vi "Main.vi"() -> ()   [LabVIEW 2020, in "Mock Temperature Controller.lvlib"]
uses:
  Mock Temperature Controller.lvlib
  process loops/Instrument Manager/Instrument State.ctl
  process loops/UI Manager/Data Display Loop Data.ctl
  process loops/Logging/Logging Configuration.ctl
  process loops/UI Manager/UI Data.ctl
  process loops/UI Manager/UI Display State.ctl
  Typedefs/System Control Data.ctl
  <vilib>/Utility/error.llb/Error Cluster From Error Code.vi
  <vilib>/ErrorRing/Error Ring.xnode
  support/Message Queue/Message Queue.lvlib
  support/User Event - Stop/User Event - Stop.lvlib
  process loops/Instrument Manager/Instrument Manager.lvlib
  process loops/Acquisition/Acquisition.lvlib
  process loops/Remote Connection Manager/Remote Connection Manager.lvlib
  process loops/Logging/Logging.lvlib
panel:
  in  "Time Interval (sec)":i32=1200
  out "Temperature Graph":cluster{timestamp[], dbl[]}[](graph)
  in  "Config Log Btn":bool
  in  "Sampling rate\n(sec/sample)":dbl=1.0 min=0.1 step=0.1
  in  "Log Data":bool
  in  "Stop Btn":bool=TRUE
  in  "Run Btn":bool
  out "Temperature Ind":dbl format="%.3f °C"
  in  "Setpoint":dbl format="%.3f °C"
  out "VISA resource":refnum<visa-resource-name>
  # "Mock Temperature Controller"
  # "Config"
  # "Instrument Control"
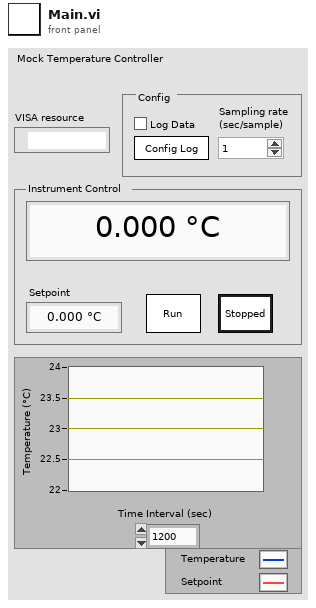
[diagram p1: front panel]
types:
  T1 = typedef "Mock Temperature Controller.lvlib/Data Display Loop Data.ctl" = cluster{"Data Timestamps":timestamp[], "Data Values":dbl[], "Setpoint":dbl[], "Previous Run State":bool}
  T2 = typedef "Mock Temperature Controller.lvlib/Instrument Manager.lvlib/Instrument State.ctl" = cluster{"VISA Resource":refnum<visa-resource-name>, "Setpoint":dbl, "Running":bool, "Running Since":timestamp, "Data Point":cluster{"Time Stamp":timestamp, "Value":dbl}, "Current Temperature":dbl, "Sampling Rate (sec/sample)":dbl}
  T3 = typedef "Mock Temperature Controller.lvlib/Message Queue.lvlib/All Message Queues.ctl" = cluster{"System Control":refnum<queue>, "Instrument":refnum<queue>, "Remote":refnum<queue>, "UI":refnum<queue>, "Acquisition":refnum<queue>, "Logging":refnum<queue>}
  T4 = typedef "Mock Temperature Controller.lvlib/UI Display State.ctl" = enum16{"Shown", "Hidden"}
  T5 = enum8{"Enabled", "Disabled", "Disabled and Grayed Out"}
  T6 = typedef "Mock Temperature Controller.lvlib/UI Data.ctl" = cluster{"VISA Resource Ind":refnum<vi>, "Setpoint Ctl":refnum<vi>, "Run Btn":refnum<vi>, "Stop Btn":refnum<vi>, "Temperature Ind":refnum<vi>, "Log Data":refnum<vi>, "Config Log Btn":refnum<vi>, "Sampling rate\n(sec/sample)":refnum<vi>, "Temperature Graph":refnum<vi>}
  T7 = typedef "Mock Temperature Controller.lvlib/Logging.lvlib/Logging Configuration.ctl" = cluster{"Log Directory Path":path, "Log File Path":path, "Log File Prefix":string, "Log File Extension":string, "File Delimiter":string, "Header Info":string[][], "Channels":string[], "Log Instrument Runs":bool}
  T8 = typedef "Mock Temperature Controller.lvlib/System Control Data.ctl" = cluster{"Example Value <Replace Me>":dbl, "Log Runs":bool, "Clone":bool}
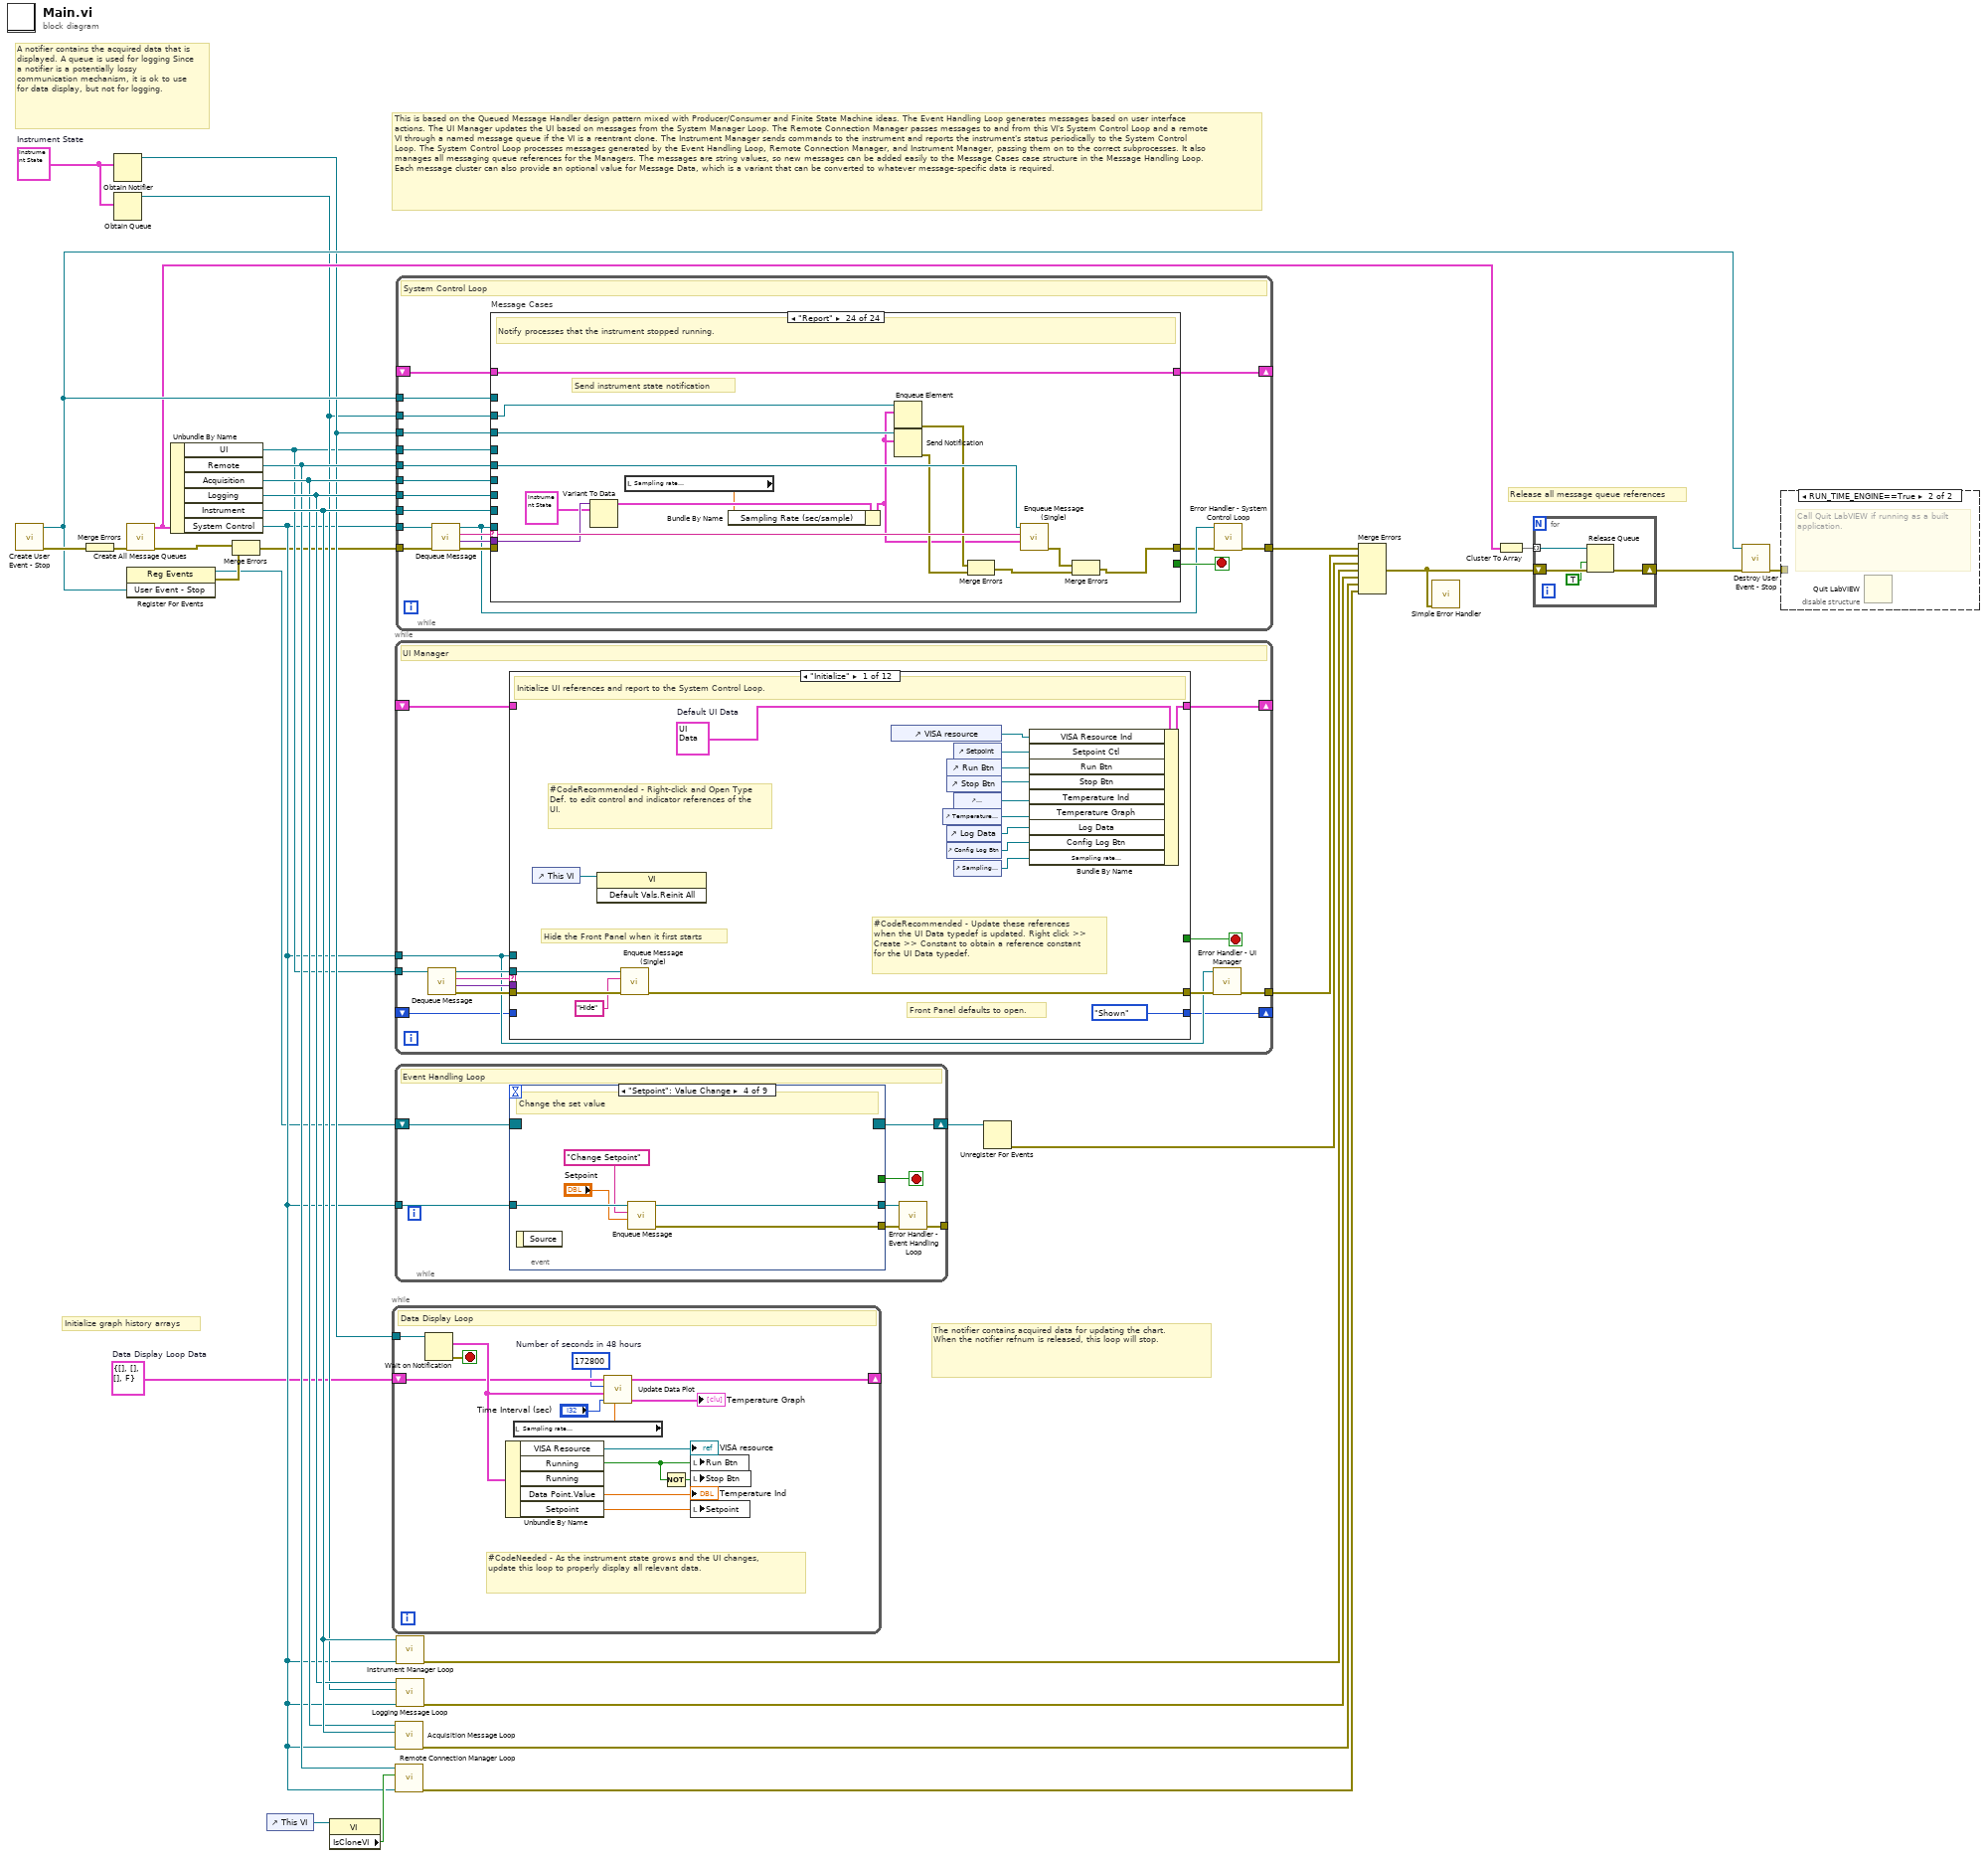
[diagram p0: block diagram]
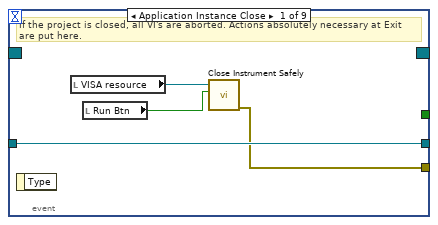
[diagram p2: hidden frame]
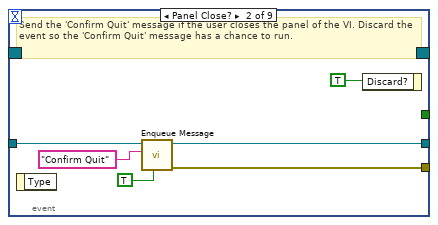
[diagram p3: hidden frame]
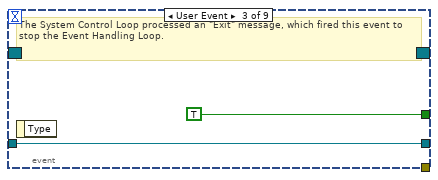
[diagram p4: hidden frame]
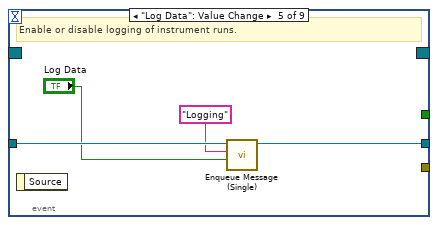
[diagram p5: hidden frame]
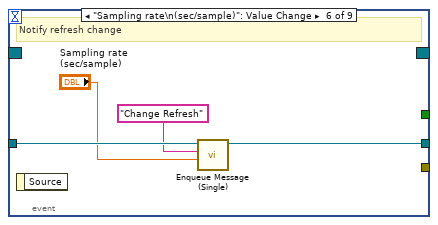
[diagram p6: hidden frame]
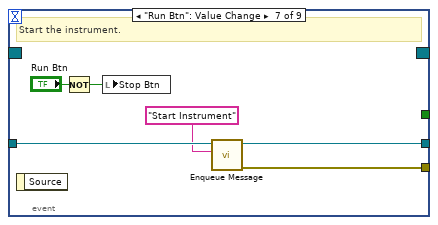
[diagram p7: hidden frame]
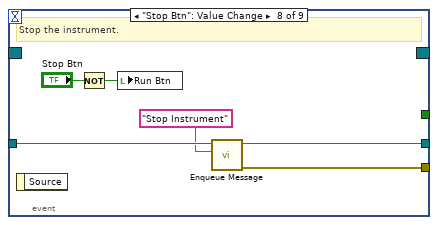
[diagram p8: hidden frame]
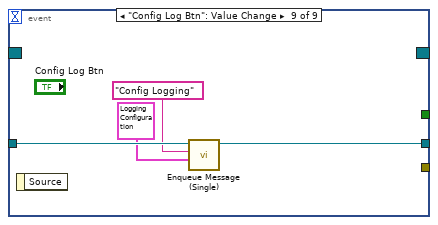
[diagram p9: hidden frame]
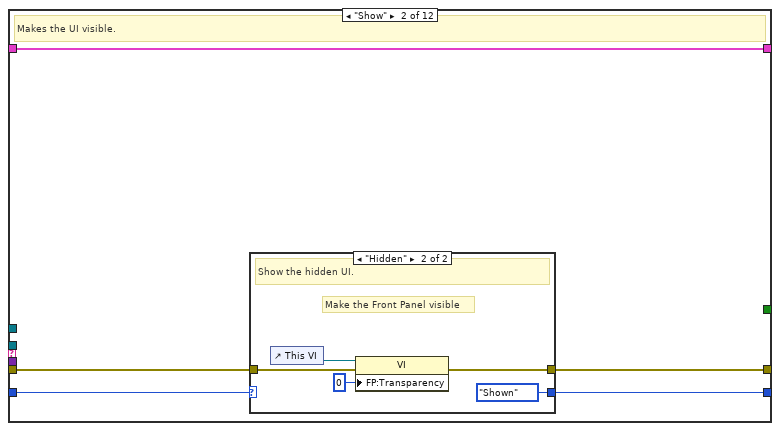
[diagram p10: hidden frame]
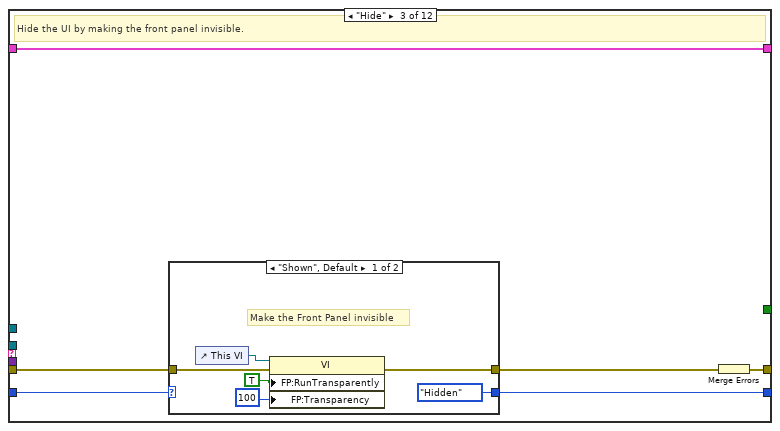
[diagram p12: hidden frame]
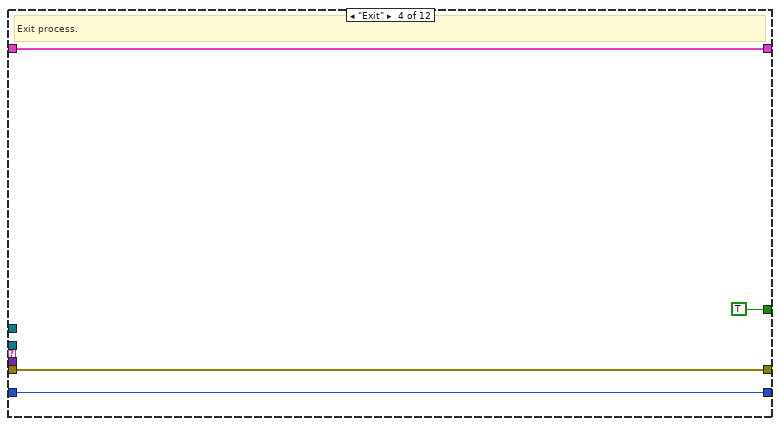
[diagram p14: hidden frame]
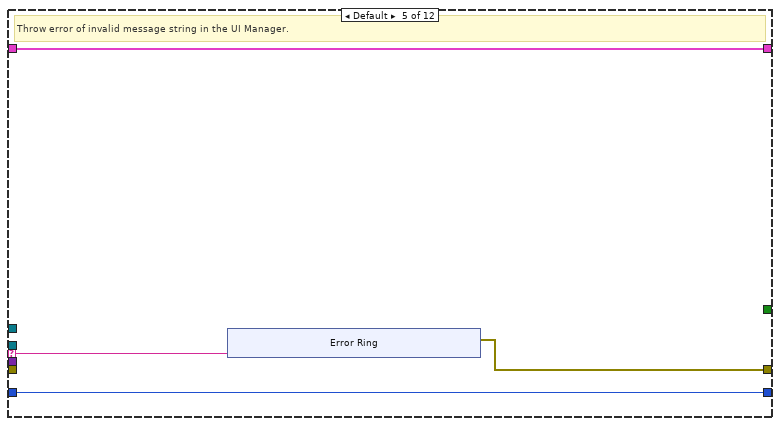
[diagram p15: hidden frame]
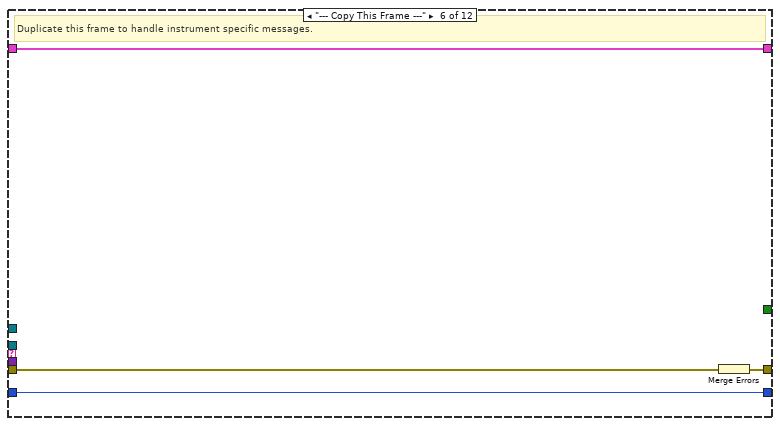
[diagram p16: hidden frame]
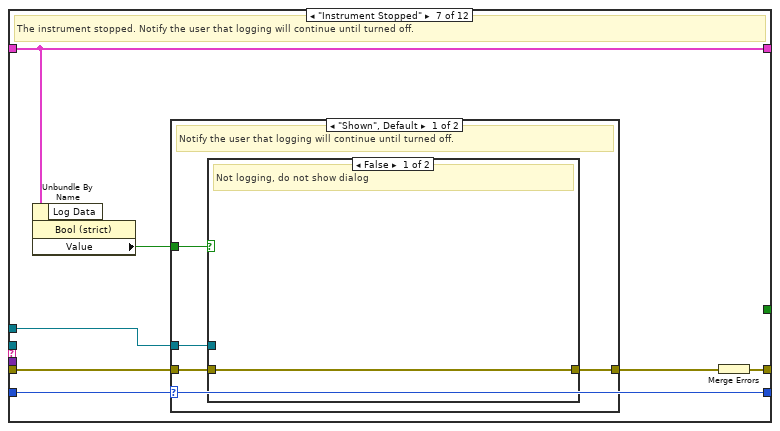
[diagram p17: hidden frame]
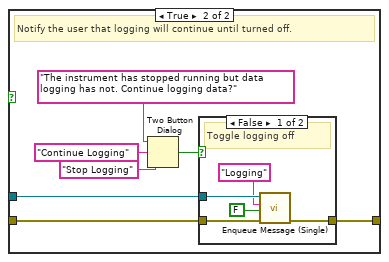
[diagram p18: hidden frame]
diagram:
  w1 = T1 {"Data Timestamps"=[], "Data Values"=[], "Setpoint"=[], "Previous Run State"=FALSE}  # Data Display Loop Data
  w7 = T2 {"VISA Resource"="", "Setpoint"=0.0, "Running"=FALSE, "Running Since"=timestamp(0 s since 1904-01-01), "Data Point"={"Time Stamp"=timestamp(0 s since 1904-01-01), "Value"=0.0}, "Current Temperature"=0.0, "Sampling Rate (sec/sample)"=0.0}  # Instrument State
  # "Initialize graph history arrays"
  # "A notifier contains the acquired data that is displayed. A queue is used for logging Since a notifier is a potentially lossy communication mechanism, it is ok to use for data display, but not for logging."
  # "The notifier contains acquired data for updating the chart. When the notifier refnum is released, this loop will stop."
  # "Release all message queue references"
  # "This is based on the Queued Message Handler design pattern mixed with Producer/Consumer and Finite State Machine ideas. The Event Handling Loop generates messages based on user interface actions. The UI Manager updates the UI based on messages from the System Manager Loop. The Remote Connection Manager passes messages to and from this VI's System Control Loop and a remote VI through a named message queue if the VI is a reentrant clone. The Instrument Manager sends commands to the instrument and reports the instrument's status periodically to the System Control Loop. The System Control Loop processes messages generated by the Event Handling Loop, Remote Connection Manager, and Instrument Manager, passing them on to the correct subprocesses. It also manages all messaging queue references for the Managers. The messages are string values, so new messages can be added easily to the Message Cases case structure in the Message Handling Loop.  Each message cluster can also provide an optional value for Message Data, which is a variant that can be converted to whatever message-specific data is required."
  n1 = call "Create User Event - Stop.vi"() -> ("error out"=w26:errorcluster, "User Event - Stop"=w22:refnum<user-event>)  [unwired: 10 in]
  n2 = Merge Errors(w26) -> (w25:errorcluster)
  n3 = Obtain Notifier(notification data type=w7) -> (notifier out=w8:refnum<notifier>)  [unwired: 3 in, 2 out]
  n4 = Obtain Queue(element data type=w7) -> (queue out=w6:refnum<queue>)  [unwired: 4 in, 2 out]
  n5 = call "Create All Message Queues.vi"("error in (no error)"=w25) -> ("error out"=w28:errorcluster, "Message Queues out"=w11:T3)  [unwired: 9 in]
  n6 = register-events(w22) -> (reference out=w2:refnum<event-registration>, error out=w13:errorcluster)  [unwired: 2 in]
  n7 = Unbundle By Name(w11) -> ("UI"=w5:refnum<queue>, "Remote"=w29:refnum<queue>, "Acquisition"=w30:refnum<queue>, "Logging"=w31:refnum<queue>, "Instrument"=w32:refnum<queue>, "System Control"=w4:refnum<queue>)
  n8 = Merge Errors(w28, w13) -> (w3:errorcluster)
  n9 = control-ref of="This VI"() -> (w21:refnum<vi>)
  n10 = property class="VI"(reference=w21) -> ("IsCloneVI"=w20:bool)  [unwired: 1 in, 2 out]
  n11 = while "Data Display Loop" {
    tunnel: w8 -> [w46]
    shift-right: [w36] -> _
    shift-left: w1 -> [w37]
    stop <- w45 stop-if-true
    w33 = 172800  # Number of seconds in 48 hours
    # "#CodeNeeded - As the instrument state grows and the UI changes, update this loop to properly display all relevant data."
    # "Data Display Loop"
    n12 = Wait on Notification(notifier=w46) -> (notification=w38:T2, error out=w45:errorcluster)  [unwired: 3 in, 2 out]
    n13 = Unbundle By Name(w38) -> ("VISA Resource"=→"VISA resource":refnum<visa-resource-name>, "Running"=w43:bool, "Data Point.Value"=→"Temperature Ind":dbl, "Setpoint"=w40:dbl)  [unwired: 1 out]
    n14 = local read "Sampling rate\n(sec/sample)"() -> (w34:dbl)
    n15 = call "Update Data Plot.vi"("Sample Rate (sec/sample)"=w34, "Time interval (s)"="Time Interval (sec)", "Instrument State"=w38, "History length"=w33, "Graph History Arrays in"=w37) -> ("Updated Plot History"=→"Temperature Graph":cluster{timestamp[], dbl[]}[], "Graph History Arrays out"=w36:T1)  [unwired: 5 in]
    n16 = Not(x=w43) -> (.not. x?=w42:bool)
    n17 = local write "Run Btn"(w43) -> ()
    n18 = local write "Stop Btn"(w42) -> ()
    n19 = local write "Setpoint"(w40) -> ()
  }
  n20 = while {
    tunnel: w5 -> [w59]
    tunnel: w4 -> [w50]
    tunnel: [w51] -> w19
    shift-right: [w54] -> _
    shift-left: _ -> [w53]
    shift-right: [w48] -> _
    shift-left: _ -> [w47]
    stop <- w49 stop-if-true
    # "UI Manager"
    n21 = call "Dequeue Message.vi"("Message Queue"=w59) -> ("error out"=w57:errorcluster, "Message Data"=w55:variant, "Message"=w56:string, "dup Message Queue"=w58:refnum<queue>)  [unwired: 7 in]
    n22 = case shown="\"Initialize\"" w56 {
      selector: w56 -> [_ _ _ _ w110 _ _ _ _ _ _ _]
      tunnel: w58 -> [w67 _ _ _ _ _ _ _ _ _ _ _]
      tunnel: w57 -> [w73 w80 w92 w106 _ w119 w127 w155 w163 w171 w182 w193]
      tunnel: w55 -> [_ _ _ _ _ _ _ _ _ w170 w180 w191]
      tunnel: w50 -> [_ _ _ _ _ _ w125 _ _ _ _ _]
      tunnel: [w68 w79 w93 w106 w109 w120 w129 w156 w164 w172 w183 w194] -> w52
      tunnel: [w75 w81 w94 w105 w108 w121 w124 w151 w157 w166 w174 w185] -> w54
      tunnel: w53 -> [_ w81 w94 w105 w108 w121 w124 w151 w157 w166 w174 w185]
      tunnel: [_ _ _ TRUE _ _ _ _ _ _ _ _] -> w49
      tunnel: w47 -> [_ w78 w90 w103 w107 w118 w128 w154 w162 w168 w175 w186]
      tunnel: [UI_Display_State."Shown" ("UI Display State") w77 w89 w103 w107 w118 w128 w154 w162 w168 w175 w186] -> w48
      frame "Initialize" {
        w76 = T6 {"VISA Resource Ind"=refnum, "Setpoint Ctl"=refnum, "Run Btn"=refnum, "Stop Btn"=refnum, "Temperature Ind"=refnum, "Log Data"=refnum, "Config Log Btn"=refnum, "Sampling rate\n(sec/sample)"=refnum, "Temperature Graph"=refnum}  # Default UI Data
        # "Front Panel defaults to open."
        # "Hide the Front Panel when it first starts"
        # "#CodeRecommended - Update these references when the UI Data typedef is updated. Right click >> Create >> Constant to obtain a reference constant for the UI Data typedef."
        # "#CodeRecommended - Right-click and Open Type Def. to edit control and indicator references of the UI."
        # "Initialize UI references and report to the System Control Loop."
        n23 = control-ref of="This VI"() -> (w60:refnum<vi>)
        n24 = invoke class="VI" method="Default Vals.Reinit All"(reference=w60) -> ()  [unwired: 2 in, 3 out]
        n25 = call "Enqueue Message (Single).vi"("error in (no error)"=w73, "Message"="Hide", "Message Queue"=w67) -> ("error out"=w68:errorcluster)  [unwired: 7 in, 1 out]
        n26 = control-ref of="VISA resource"() -> (w72:refnum<vi>)
        n27 = control-ref of="Temperature Graph"() -> (w64:refnum<vi>)
        n28 = control-ref of="Run Btn"() -> (w70:refnum<vi>)
        n29 = control-ref of="Stop Btn"() -> (w71:refnum<vi>)
        n30 = control-ref of="Log Data"() -> (w63:refnum<vi>)
        n31 = control-ref of="Config Log Btn"() -> (w62:refnum<vi>)
        n32 = control-ref of="Setpoint"() -> (w74:refnum<vi>)
        n33 = control-ref of="Temperature Ind"() -> (w69:refnum<vi>)
        n34 = control-ref of="Sampling rate (sec/sample)"() -> (w61:refnum<vi>)
        n35 = Bundle By Name(cluster=w76, "VISA Resource Ind"=w72, "Setpoint Ctl"=w74, "Run Btn"=w70, "Stop Btn"=w71, "Temperature Ind"=w69, "Temperature Graph"=w64, "Log Data"=w63, "Config Log Btn"=w62, "Sampling rate\n(sec/sample)"=w61) -> (w75:T6)
      }
      frame "Show" {
        # "Makes the UI visible."
        n36 = case shown="\"Hidden\"" w78 {
          selector: w78 -> [w83 _]
          tunnel: w80 -> [w82 w88]
          tunnel: [w82 w86] -> w79
          tunnel: [w83 UI_Display_State."Shown" ("UI Display State")] -> w77
          frame "Shown", Default {
            # "Do nothing if UI is already shown."
          }
          frame "Hidden" {
            # "Make the Front Panel visible"
            # "Show the hidden UI."
            n37 = control-ref of="This VI"() -> (w87:refnum<vi>)
            n38 = property class="VI"(reference=w87, error in=w88, "FP:Transparency"=u8 0 ("Front Panel Window:Transparency")) -> (error out=w86:errorcluster)  [unwired: 1 out]
          }
        }
      }
      frame "Hide" {
        # "Hide the UI by making the front panel invisible."
        n39 = case shown="\"Shown\", Default" w90 {
          selector: w90 -> [_ w102]
          tunnel: w92 -> [w97 w101]
          tunnel: [w96 w101] -> w91
          tunnel: [UI_Display_State."Hidden" ("UI Display State") w102] -> w89
          frame "Shown", Default {
            # "Make the Front Panel invisible"
            n40 = control-ref of="This VI"() -> (w100:refnum<vi>)
            n41 = property class="VI"(reference=w100, error in=w97, "FP:RunTransparently"=TRUE ("Front Panel Window:Run VI Transparently"), "FP:Transparency"=u8 100 ("Front Panel Window:Transparency")) -> (error out=w96:errorcluster)  [unwired: 1 out]
          }
          frame "Hidden" {
          }
        }
        n42 = Merge Errors(w91) -> (w93:errorcluster)
      }
      frame "Exit" {
        # "Exit process."
      }
      frame Default {
        # "Throw error of invalid message string in the UI Manager."
        n43 = xnode "Error Ring"("parameter 0"=w110) -> ("error out"=w109:errorcluster)
      }
      frame "--- Copy This Frame ---" {
        # "Duplicate this frame to handle instrument specific messages."
        n44 = Merge Errors(w119) -> (w120:errorcluster)
      }
      frame "Instrument Stopped" {
        # "The instrument stopped. Notify the user that logging will continue until turned off."
        n45 = Unbundle By Name(w124) -> ("Log Data"=w123:refnum<vi>)
        n46 = property class="Bool (strict)"(reference=w123) -> ("Value"=w122:bool)  [unwired: 1 in, 2 out]
        n47 = case shown="\"Shown\", Default" w128 {
          tunnel: w127 -> [w133 w148]
          tunnel: [w132 w148] -> w126
          tunnel: w125 -> [w131 _]
          tunnel: w122 -> [w130 _]
          frame "Shown", Default {
            # "Notify the user that logging will continue until turned off."
            n48 = case shown="False" w130 {
              tunnel: w133 -> [w134 w137]
              tunnel: [w134 w136] -> w132
              tunnel: w131 -> [_ w135]
              frame False {
                # "Not logging, do not show dialog"
              }
              frame True {
                # "Notify the user that logging will continue until turned off."
                n49 = Two Button Dialog(message="The instrument has stopped running but data logging has not. Continue logging data?", 1:"Stop Logging" ("F button name (\"Cancel\")"), 2:"Continue Logging" ("T button name (\"OK\")")) -> (T button?=w138:bool)
                n50 = case shown="False" w138 {
                  tunnel: w137 -> [w146 w147]
                  tunnel: [w145 w147] -> w136
                  tunnel: w135 -> [w144 _]
                  frame False {
                    # "Toggle logging off"
                    n51 = call "Enqueue Message (Single).vi"("error in (no error)"=w146, "Message Data"=FALSE, "Message"="Logging", "Message Queue"=w144) -> ("error out"=w145:errorcluster)  [unwired: 6 in, 1 out]
                  }
                  frame True {
                    # "Continues logging. Do nothing more"
                  }
                }
              }
            }
          }
          frame "Hidden" {
            # "Hidden, do not show dialog"
          }
        }
        n52 = Merge Errors(w126) -> (w129:errorcluster)
      }
      frame "Logging Started" {
        # "Indicate that logging started."
        n53 = Unbundle By Name(w151) -> ("Log Data"=w153:refnum<vi>)
        n54 = property class="Bool (strict)"(reference=w153, "Value"=TRUE ("Log Data")) -> ()  [unwired: 1 in, 2 out]
        n55 = Unbundle By Name(w151) -> ("Config Log Btn"=w150:refnum<vi>)
        n56 = property class="Bool"(reference=w150, "DisabledEnum"=T5."Disabled and Grayed Out" ("Disabled")) -> ()  [unwired: 1 in, 2 out]
        n57 = Merge Errors(w155) -> (w156:errorcluster)
      }
      frame "Logging Stopped" {
        # "Indicate that logging stopped."
        n58 = Unbundle By Name(w157) -> ("Log Data"=w161:refnum<vi>)
        n59 = property class="Bool (strict)"(reference=w161, "Value"=FALSE ("Log Data")) -> ()  [unwired: 1 in, 2 out]
        n60 = Unbundle By Name(w157) -> ("Config Log Btn"=w159:refnum<vi>)
        n61 = property class="Bool"(reference=w159, "DisabledEnum"=T5."Enabled" ("Disabled")) -> ()  [unwired: 1 in, 2 out]
        n62 = Merge Errors(w163) -> (w164:errorcluster)
      }
      frame "Change Refresh" {
        # "Update sample rate multiplier in the UI data chart and config indicator."
        n63 = Unbundle By Name(w166) -> ("Sampling rate\n(sec/sample)"=w167:refnum<vi>)
        n64 = Variant To Data(type=0.0, Variant=w170) -> (data=w165:dbl)  [unwired: 1 in, 1 out]
        n65 = property class="DigNum (strict)"(reference=w167, "Value"=w165) -> ()  [unwired: 1 in, 2 out]
        n66 = Merge Errors(w171) -> (w172:errorcluster)
      }
      frame "Display Units - Temperature Ind" {
        # "#CodeRecommended - If this format string is changed, update it on the front panel indicator as well."
        # "Change the units of the display."
        n67 = Variant To Data(type="", Variant=w180) -> (data=w178:string)  [unwired: 1 in, 1 out]
        n68 = call <vilib>:"Space Constant.vi"() -> ("String"=w179:string)
        n69 = Concatenate Strings("%.3f" ("string"), w179, w178) -> (w176:string)
        n70 = Unbundle By Name(w174) -> ("Temperature Ind"=w173:refnum<vi>)
        n71 = property on="Property Node" class="DigNum (strict)"(reference=w173, "FormatString"=w176) -> ()  [unwired: 1 in, 2 out]
        n72 = Merge Errors(w182) -> (w183:errorcluster)
      }
      frame "Display Units - Setpoint" {
        # "#CodeRecommended - If this format string is changed, update it on the front panel indicator as well."
        # "Change the units of the setpoint display."
        n73 = Variant To Data(type="", Variant=w191) -> (data=w189:string)  [unwired: 1 in, 1 out]
        n74 = call <vilib>:"Space Constant.vi"() -> ("String"=w190:string)
        n75 = Concatenate Strings("%.3f" ("string"), w190, w189) -> (w187:string)
        n76 = Unbundle By Name(w185) -> ("Setpoint Ctl"=w184:refnum<vi>)
        n77 = property on="Property Node" class="DigNum (strict)"(reference=w184, "FormatString"=w187) -> ()  [unwired: 1 in, 2 out]
        n78 = Merge Errors(w193) -> (w194:errorcluster)
      }
    }
    n79 = call "Error Handler - UI Manager.vi"("error in (no error)"=w52, "Message Queue"=w50) -> ("dup error in"=w51:errorcluster)  [unwired: 8 in, 1 out]
  }
  n80 = while {
    tunnel: w4 -> [w201]
    shift-right: [w199] -> w23
    shift-left: w2 -> [w200]
    tunnel: [w195] -> _
    stop <- w197 stop-if-true
    # "Event Handling Loop"
    n81 = event shown="[3] \"Setpoint\": Value Change" {
      selector: w200 -> [_ _ _ _ _ _ _ _ _]
      dyn-events: [_ _ _ _ _ _ _ _ _] -> w199
      timeout: _ -> [_ _ _ _ _ _ _ _ _]
      tunnel: [_ _ TRUE ("Discard?") _ _ _ _ _ _] -> w197
      tunnel: w201 -> [w205 w210 w213 w218 w222 w226 w232 w238 w242]
      tunnel: [w204 w209 _ w215 _ _ w230 w236 _] -> w198
      tunnel: [w205 w208 w213 w217 w221 w225 w231 w237 w241] -> w196
      event Application Instance Close {
        # "If the project is closed, all VI's are aborted. Actions absolutely necessary at Exit are put here."
        n82 = event-data() -> ()  [unwired: 1 in, 1 out]
        n83 = local read "VISA resource"() -> (w203:refnum<visa-resource-name>)
        n84 = local read "Run Btn"() -> (w202:bool)
        n85 = call "Close Instrument Safely.vi"("Running (F)"=w202, "VISA Refnum in"=w203) -> ("error out"=w204:errorcluster)  [unwired: 9 in]
      }
      event Panel Close? {
        # "Send the 'Confirm Quit' message if the user closes the panel of the VI. Discard the event so the 'Confirm Quit' message has a chance to run."
        n86 = event-data() -> ()  [unwired: 1 in, 1 out]
        n87 = call-poly "Enqueue Message.vi"("Priority Message? (F)"=TRUE, "Message"="Confirm Quit", "Message Queue"=w210) -> ("error out"=w209:errorcluster, "dup Message Queue"=w208:refnum<queue>)  [unwired: 7 in]
        n88 = event-data("Discard?"=TRUE) -> ()  [unwired: 1 in, 1 out]
      }
      event User Event {
        # "The System Control Loop processed an \"Exit\" message, which fired this event to stop the Event Handling Loop."
        n89 = event-data() -> ()  [unwired: 1 in, 1 out]
      }
      event "Setpoint": Value Change {
        # "Change the set value"
        n90 = event-data() -> ()  [unwired: 1 in, 1 out]
        n91 = call-poly "Enqueue Message.vi"("Message Data"="Setpoint", "Message"="Change Setpoint", "Message Queue"=w218) -> ("error out"=w215:errorcluster, "dup Message Queue"=w217:refnum<queue>)  [unwired: 7 in]
      }
      event "Log Data": Value Change {
        # "Enable or disable logging of instrument runs."
        n92 = event-data() -> ()  [unwired: 1 in, 1 out]
        n93 = call "Enqueue Message (Single).vi"("Message Data"="Log Data", "Message"="Logging", "Message Queue"=w222) -> ("dup Message Queue"=w221:refnum<queue>)  [unwired: 7 in, 1 out]
      }
      event "Sampling rate\n(sec/sample)": Value Change {
        # "Notify refresh change"
        n94 = event-data() -> ()  [unwired: 1 in, 1 out]
        n95 = call "Enqueue Message (Single).vi"("Message Data"="Sampling rate\n(sec/sample)", "Message"="Change Refresh", "Message Queue"=w226) -> ("dup Message Queue"=w225:refnum<queue>)  [unwired: 7 in, 1 out]
      }
      event "Run Btn": Value Change {
        # "Start the instrument."
        n96 = event-data() -> ()  [unwired: 1 in, 1 out]
        n97 = Not(x="Run Btn") -> (.not. x?=w227:bool)
        n98 = local write "Stop Btn"(w227) -> ()
        n99 = call-poly "Enqueue Message.vi"("Message"="Start Instrument", "Message Queue"=w232) -> ("error out"=w230:errorcluster, "dup Message Queue"=w231:refnum<queue>)  [unwired: 8 in]
      }
      event "Stop Btn": Value Change {
        # "Stop the instrument."
        n100 = event-data() -> ()  [unwired: 1 in, 1 out]
        n101 = Not(x="Stop Btn") -> (.not. x?=w233:bool)
        n102 = local write "Run Btn"(w233) -> ()
        n103 = call-poly "Enqueue Message.vi"("Message"="Stop Instrument", "Message Queue"=w238) -> ("error out"=w236:errorcluster, "dup Message Queue"=w237:refnum<queue>)  [unwired: 8 in]
      }
      event "Config Log Btn": Value Change {
        n104 = event-data() -> ()  [unwired: 1 in, 1 out]
        n105 = call "Enqueue Message (Single).vi"("Message Data"=T7 {"Log Directory Path"=path "", "Log File Path"=path "", "Log File Prefix"="Experiment", "Log File Extension"="csv", "File Delimiter"=",", "Header Info"=[], "Channels"=[], "Log Instrument Runs"=FALSE} ("Logging Configuration"), "Message"="Config Logging", "Message Queue"=w242) -> ("dup Message Queue"=w241:refnum<queue>)  [unwired: 7 in, 1 out]
      }
    }
    n106 = call "Error Handler - Event Handling Loop.vi"("error in (no error)"=w198, "Message Queue"=w196) -> ("dup error in"=w195:errorcluster)  [unwired: 8 in, 1 out]
  }
  n107 = call "Acquisition Message Loop.vi"("System Control"=w4, "Instrument Manager"=w32, "Acquisition"=w30) -> ("error out"=w15:errorcluster)  [unwired: 8 in]
  n108 = call "Remote Connection Manager Loop.vi"("System Control"=w4, "IsCloneVI (false)"=w20, "RCM Queue"=w29) -> ("error out"=w14:errorcluster)  [unwired: 8 in]
  n109 = while {
    tunnel: w4 -> [w253]
    shift-right: [w260] -> _
    shift-left: _ -> [w261]
    tunnel: w22 -> [w258]
    tunnel: w3 -> [w257]
    tunnel: [w251] -> w27
    tunnel: w32 -> [w249]
    tunnel: w29 -> [w248]
    tunnel: w5 -> [w247]
    tunnel: w30 -> [w246]
    tunnel: w31 -> [w245]
    tunnel: w8 -> [w244]
    tunnel: w6 -> [w243]
    stop <- w259 stop-if-true
    # "System Control Loop"
    n110 = call "Dequeue Message.vi"("error in (no error)"=w257, "Message Queue"=w253) -> ("error out"=w256:errorcluster, "Message Data"=w254:variant, "Message"=w255:string, "dup Message Queue"=w252:refnum<queue>)  [unwired: 6 in]
    n111 = case "Message Cases" shown="\"Report\"" w255 {
      selector: w255 -> [_ _ _ w303 w316 w327 w345 w359 w365 _ w411 w418 w425 w432 w439 w449 w463 w478 w492 w503 w510 w520 w535 w557]
      tunnel: w252 -> [_ _ w283 _ _ _ _ _ _ _ _ _ _ _ _ _ _ _ _ _ _ _ _ _]
      tunnel: w256 -> [w265 w280 w287 _ _ w330 w348 w363 w381 w394 w415 w422 w429 w436 w443 w452 w466 w482 w496 w506 w513 _ _ _]
      tunnel: [w264 w274 w285 w306 w317 w336 w350 w364 w372 w399 w416 w423 w430 w437 w444 w453 w467 w480 w494 w507 w514 w519 w534 w556] -> w250
      tunnel: w261 -> [_ w279 w286 w302 w318 w337 w351 w362 w371 w400 w417 w424 w431 w438 w445 w454 w468 w481 w495 w508 w515 w518 w531 w554]
      tunnel: [w266 w279 w286 w302 w318 w337 w351 w362 w371 w398 w417 w424 w431 w438 w445 w454 w468 w481 w495 w508 w515 w518 w531 w554] -> w260
      tunnel: [_ _ _ TRUE _ _ _ _ _ _ _ _ _ _ _ _ _ _ _ _ _ _ _ _] -> w259
      tunnel: w254 -> [_ w278 _ w307 _ w326 w344 w358 w366 w396 w412 w419 w426 w433 w440 w450 w464 w477 w491 w504 w511 w521 w536 w552]
      tunnel: w258 -> [_ _ _ w304 _ _ _ _ _ _ _ _ _ _ _ _ _ _ _ _ _ _ _ _]
      tunnel: w249 -> [w263 _ _ w299 _ w331 _ w360 _ _ _ _ _ _ _ _ _ _ w490 w502 w509 _ _ _]
      tunnel: w248 -> [_ _ _ w298 _ w334 w349 _ w376 _ _ _ _ _ _ w448 w462 _ _ _ _ w522 w532 w555]
      tunnel: w247 -> [_ _ _ w297 _ w333 _ _ w375 _ _ _ _ _ _ w447 w461 w475 _ _ _ _ w530 _]
      tunnel: w246 -> [_ _ _ w301 _ w335 _ _ w378 _ _ _ _ _ _ _ _ w476 w489 _ _ w517 _ _]
      tunnel: w245 -> [_ _ _ w300 _ w332 _ _ w368 w392 w413 w420 w427 w434 w441 _ _ _ _ _ _ w516 _ _]
      tunnel: w244 -> [_ _ _ w294 _ _ _ _ _ _ _ _ _ _ _ _ _ _ _ _ _ _ _ w553]
      tunnel: w243 -> [_ _ _ w292 _ _ _ _ _ _ _ _ _ _ _ _ _ _ _ _ _ _ _ w549]
      frame "Initialize" {
        w267 = T8 {"Example Value <Replace Me>"=0.0, "Log Runs"=FALSE, "Clone"=FALSE}  # Default Data
        # "Initialize the system control loop and system."
        n112 = control-ref of="This VI"() -> ()  [unwired: 1 out]
        n113 = property on="Property Node" class="VI"() -> ("IsCloneVI"=w262:bool)  [unwired: 2 in, 2 out]
        n114 = Bundle By Name(cluster=w267, "Clone"=w262) -> (w266:T8)
        n115 = case shown="False" w262 {
          tunnel: w265 -> [w270 w273]
          tunnel: [w269 w273] -> w264
          tunnel: w263 -> [w268 _]
          frame False {
            # "Initiate the VISA Resource selection window if this is not a"
            n116 = call "Enqueue Message (Single).vi"("error in (no error)"=w270, "Message Data"=refnum<visa-resource-name> refnum ("VISA resource out"), "Message"="Set VISA Resource", "Message Queue"=w268) -> ("error out"=w269:errorcluster)  [unwired: 6 in, 1 out]
          }
          frame True {
            # "Reentrant clone. It is the responsibility of the RCM to send the Set VISA Resource command."
          }
        }
      }
      frame "Error" {
        # "#CodeRecommended - If you ever change the name of this \"Error\" message, you'll need to update the name in the Check Loop Error.vi as well."
        # "#CodeRecommended - Consider creating a system for logging errors in some way. These errors are for notification purposes only. Handling of specific errors should be performed in the message frames that generated the error."
        # "Error - Display an error dialog. This message is sent by the \"Error Handler\" VIs at the end of other loops in this application."
        n117 = Variant To Data(error in=w280, type=errorcluster {"status"=FALSE, "code"=0, "source"=""} ("error constant"), Variant=w278) -> (data=w276:errorcluster, error out=w275:errorcluster)
        n118 = call <vilib>:"Simple Error Handler.vi"("error in (no error)"=w276) -> ()  [unwired: 4 in, 5 out]
        n119 = Merge Errors(w275) -> (w274:errorcluster)
      }
      frame "Confirm Quit" {
        # "#CodeNeeded - If you want to provide an \"Are you sure\" dialog (or some other notification) before the application exits, place that code here. This message is typically sent from a Panel Close? event."
        # "Confirm Quit - Message that can confirm whether or not the user wants to exit the application."
        n120 = call-poly "Enqueue Message.vi"("Priority Message? (F)"=TRUE, "error in (no error)"=w287, "Message"="Exit", "Message Queue"=w283) -> ("error out"=w284:errorcluster)  [unwired: 6 in, 1 out]
        n121 = Merge Errors(w284) -> (w285:errorcluster)
      }
      frame "Exit" {
        # "Order other processes to exit"
        # "Begin the application closing procedure by sending \"Exit\" commands to all running processes."
        n122 = Variant To Data(type=errorcluster {"status"=FALSE, "code"=0, "source"=""} ("error constant"), Variant=w307) -> (data=w308:errorcluster)  [unwired: 1 in, 1 out]
        n123 = Build Array(w297, w298, w301, w300, w299) -> (w296:refnum<queue>[])
        n124 = call <vilib>:"Clear Errors.vi"("error in (no error)"=w308, "specific error code to clear (0: all)"=5000) -> ("error out"=w289:errorcluster)  [unwired: 4 in, 1 out]
        n125 = call <vilib>:"Simple Error Handler.vi"("error in (no error)"=w289) -> ()  [unwired: 4 in, 5 out]
        n126 = for {
          tunnel: w303 -> [w314]
          tunnel: w296 -> [w313] mode=indexing
          shift-right: [w312] -> w305
          shift-left: _ -> [w311]
          n127 = call "Enqueue Message (Single).vi"("Priority Message? (F)"=TRUE, "Message"=w314, "Message Queue"=w313) -> ("error out"=w315:errorcluster)  [unwired: 7 in, 1 out]
          n128 = Merge Errors(w315, w311) -> (w312:errorcluster)
        }
        n129 = Release Notifier(notifier=w294) -> (error out=w293:errorcluster)  [unwired: 2 in, 2 out]
        n130 = Release Queue(queue=w292) -> (error out=w290:errorcluster)  [unwired: 2 in, 2 out]
        n131 = call "Fire User Event - Stop.vi"("User Event - Stop"=w304) -> ("error out"=w291:errorcluster)  [unwired: 10 in]
        n132 = Merge Errors(w291, w290, w293, w305) -> (w306:errorcluster)
      }
      frame Default {
        # "'Default' case only runs if there is a message that isn't defined in any of the other cases.  Output a programming error."
        n133 = xnode "Error Ring"("parameter 0"=w316) -> ("error out"=w317:errorcluster)
      }
      frame "---Copy This Frame---" {
        # "Sends the message to each process in the array."
        # "#CodeRecommended - Change connections to build an array of the processes that will receive this message"
        # "Duplicate this frame when creating new messages.  Change this comment in the duplicated frame to describe this message."
        n134 = Build Array(w333, w334, w335, w332, w331) -> (w328:refnum<queue>[])
        n135 = for {
          tunnel: w328 -> [w341] mode=indexing
          tunnel: w327 -> [w343]
          tunnel: w326 -> [w342]
          shift-right: [w340] -> w329
          shift-left: w330 -> [w338]
          n136 = call "Enqueue Message (Single).vi"("Message Data"=w342, "Message"=w343, "Message Queue"=w341) -> ("error out"=w339:errorcluster)  [unwired: 7 in, 1 out]
          n137 = Merge Errors(w339, w338) -> (w340:errorcluster)
        }
        n138 = Merge Errors(w329) -> (w336:errorcluster)
      }
      frame "Set Remote Queue" {
        # "Sends the message to each process in the array."
        # "Bounce this message back to the Remote Control Manager to set the remote queue to publish messages to."
        n139 = Build Array(w349) -> (w346:refnum<queue>[])
        n140 = for {
          tunnel: w346 -> [w355] mode=indexing
          tunnel: w345 -> [w357]
          tunnel: w344 -> [w356]
          shift-right: [w354] -> w347
          shift-left: w348 -> [w352]
          n141 = call "Enqueue Message (Single).vi"("Message Data"=w356, "Message"=w357, "Message Queue"=w355) -> ("error out"=w353:errorcluster)  [unwired: 7 in, 1 out]
          n142 = Merge Errors(w353, w352) -> (w354:errorcluster)
        }
        n143 = Merge Errors(w347) -> (w350:errorcluster)
      }
      frame "Set VISA Resource" {
        # "Update the VISA Resource of the instrument."
        n144 = call "Enqueue Message (Single).vi"("error in (no error)"=w363, "Message Data"=w358, "Message"=w359, "Message Queue"=w360) -> ("error out"=w361:errorcluster)  [unwired: 6 in, 1 out]
        n145 = Merge Errors(w361) -> (w364:errorcluster)
      }
      frame "Valid VISA Resource" {
        # "When a Valid VISA Resource has been chosen, start the other processes."
        n146 = Unbundle By Name(w371) -> ("Log Runs"=w370:bool)
        n147 = call "Enqueue Message (Single).vi"("error in (no error)"=w381, "Message Data"=w366, "Message"=w365, "Message Queue"=w368) -> ("error out"=w369:errorcluster, "dup Message Queue"=w367:refnum<queue>)  [unwired: 6 in]
        n148 = case shown="True" w370 {
          tunnel: w369 -> [w382 w386]
          tunnel: w367 -> [_ w385]
          tunnel: [w382 w383] -> w379
          frame False {
          }
          frame True {
            n149 = call "Enqueue Message (Single).vi"("error in (no error)"=w386, "Message"="Start", "Message Queue"=w385) -> ("error out"=w383:errorcluster)  [unwired: 7 in, 1 out]
          }
        }
        n150 = call "Enqueue Message (Single).vi"("error in (no error)"=w379, "Message"="Start", "Message Queue"=w378) -> ("error out"=w377:errorcluster)  [unwired: 7 in, 1 out]
        n151 = Unbundle By Name(w371) -> ("Clone"=w373:bool)
        n152 = call "Enqueue Message (Single).vi"("error in (no error)"=w377, "Message Data"=w366, "Message"=w365, "Message Queue"=w376) -> ("error out"=w374:errorcluster)  [unwired: 6 in, 1 out]
        n153 = case shown="False" w373 {
          tunnel: w374 -> [w390 w391]
          tunnel: [w389 w391] -> w372
          tunnel: w375 -> [w388 _]
          frame False {
            # "Show the Front Panel automatically on startup"
            n154 = call "Enqueue Message (Single).vi"("error in (no error)"=w390, "Message"="Show", "Message Queue"=w388) -> ("error out"=w389:errorcluster)  [unwired: 7 in, 1 out]
          }
          frame True {
            # "Reentrant clone. It is the responsibility of the RCM to send \"Show\"."
          }
        }
      }
      frame "Logging" {
        # "Enable or disable logging in the System Data. Run logging is disabled by default."
        n155 = Variant To Data(type=TRUE, Variant=w396) -> (data=w395:bool)  [unwired: 1 in, 1 out]
        n156 = case shown="True" w395 {
          tunnel: w394 -> [w405 w410]
          tunnel: [w404 w409] -> w393
          tunnel: w392 -> [w403 w408]
          frame False {
            n157 = call "Enqueue Message (Single).vi"("Priority Message? (F)"=TRUE, "error in (no error)"=w405, "Message"="Stop", "Message Queue"=w403) -> ("error out"=w404:errorcluster)  [unwired: 6 in, 1 out]
          }
          frame True {
            n158 = call "Enqueue Message (Single).vi"("Priority Message? (F)"=TRUE, "error in (no error)"=w410, "Message"="Start", "Message Queue"=w408) -> ("error out"=w409:errorcluster)  [unwired: 6 in, 1 out]
          }
        }
        n159 = Bundle By Name(cluster=w400, "Log Runs"=w395) -> (w398:T8)
        n160 = Merge Errors(w393) -> (w399:errorcluster)
      }
      frame "Config Logging" {
        # "Pass on Config Logging message to Logging Loop."
        n161 = call "Enqueue Message (Single).vi"("error in (no error)"=w415, "Message Data"=w412, "Message"=w411, "Message Queue"=w413) -> ("error out"=w414:errorcluster)  [unwired: 6 in, 1 out]
        n162 = Merge Errors(w414) -> (w416:errorcluster)
      }
      frame "Set Log Directory" {
        # "Pass on log setting message to Logging Loop."
        n163 = call "Enqueue Message (Single).vi"("error in (no error)"=w422, "Message Data"=w419, "Message"=w418, "Message Queue"=w420) -> ("error out"=w421:errorcluster)  [unwired: 6 in, 1 out]
        n164 = Merge Errors(w421) -> (w423:errorcluster)
      }
      frame "Set Log File Prefix" {
        # "Pass on log setting message to Logging Loop."
        n165 = call "Enqueue Message (Single).vi"("error in (no error)"=w429, "Message Data"=w426, "Message"=w425, "Message Queue"=w427) -> ("error out"=w428:errorcluster)  [unwired: 6 in, 1 out]
        n166 = Merge Errors(w428) -> (w430:errorcluster)
      }
      frame "Set Log File Delimiter" {
        # "Pass on log setting message to Logging Loop."
        n167 = call "Enqueue Message (Single).vi"("error in (no error)"=w436, "Message Data"=w433, "Message"=w432, "Message Queue"=w434) -> ("error out"=w435:errorcluster)  [unwired: 6 in, 1 out]
        n168 = Merge Errors(w435) -> (w437:errorcluster)
      }
      frame "Set Log on Run" {
        # "Pass on log setting message to Logging Loop."
        n169 = call "Enqueue Message (Single).vi"("error in (no error)"=w443, "Message Data"=w440, "Message"=w439, "Message Queue"=w441) -> ("error out"=w442:errorcluster)  [unwired: 6 in, 1 out]
        n170 = Merge Errors(w442) -> (w444:errorcluster)
      }
      frame "Logging Started" {
        # "Pass on Logging Started message to RCM and UI."
        n171 = Build Array(w447, w448) -> (w446:refnum<queue>[])
        n172 = for {
          tunnel: w450 -> [w457]
          tunnel: w449 -> [w456]
          shift-right: [w458] -> w451
          shift-left: w452 -> [w459]
          tunnel: w446 -> [w455] mode=indexing
          n173 = call "Enqueue Message (Single).vi"("error in (no error)"=w459, "Message Data"=w457, "Message"=w456, "Message Queue"=w455) -> ("error out"=w458:errorcluster)  [unwired: 6 in, 1 out]
        }
        n174 = Merge Errors(w451) -> (w453:errorcluster)
      }
      frame "Logging Stopped" {
        # "Pass on Logging Stopped message to RCM and UI."
        n175 = Build Array(w461, w462) -> (w460:refnum<queue>[])
        n176 = for {
          tunnel: w464 -> [w471]
          tunnel: w463 -> [w470]
          shift-right: [w472] -> w465
          shift-left: w466 -> [w473]
          tunnel: w460 -> [w469] mode=indexing
          n177 = call "Enqueue Message (Single).vi"("error in (no error)"=w473, "Message Data"=w471, "Message"=w470, "Message Queue"=w469) -> ("error out"=w472:errorcluster)  [unwired: 6 in, 1 out]
        }
        n178 = Merge Errors(w465) -> (w467:errorcluster)
      }
      frame "Change Refresh" {
        # "#CodeRecommended - If the default refresh time is changed, it must be updated in the UI and Data Acquisition Loop Data typedef."
        # "Change the sampling rate of the instrument. Default is 1 second/sample."
        n179 = Build Array(w475, w476) -> (w474:refnum<queue>[])
        n180 = for {
          tunnel: w478 -> [w485]
          tunnel: w477 -> [w484]
          tunnel: w474 -> [w483] mode=indexing
          shift-right: [w486] -> w479
          shift-left: w482 -> [w487]
          n181 = call "Enqueue Message (Single).vi"("error in (no error)"=w487, "Message Data"=w484, "Message"=w485, "Message Queue"=w483) -> ("error out"=w486:errorcluster)  [unwired: 6 in, 1 out]
        }
        n182 = Merge Errors(w479) -> (w480:errorcluster)
      }
      frame "Change Setpoint" {
        # "Forward the Change Setpoint command to the IML and acquisition."
        n183 = Build Array(w489, w490) -> (w488:refnum<queue>[])
        n184 = for {
          tunnel: w492 -> [w499]
          tunnel: w491 -> [w498]
          shift-right: [w500] -> w493
          shift-left: w496 -> [w501]
          tunnel: w488 -> [w497] mode=indexing
          n185 = call "Enqueue Message (Single).vi"("error in (no error)"=w501, "Message Data"=w498, "Message"=w499, "Message Queue"=w497) -> ("error out"=w500:errorcluster)  [unwired: 6 in, 1 out]
        }
        n186 = Merge Errors(w493) -> (w494:errorcluster)
      }
      frame "Start Instrument" {
        # "Pass message to Instrument Manager Loop."
        n187 = call "Enqueue Message (Single).vi"("error in (no error)"=w506, "Message Data"=w504, "Message"=w503, "Message Queue"=w502) -> ("error out"=w505:errorcluster)  [unwired: 6 in, 1 out]
        n188 = Merge Errors(w505) -> (w507:errorcluster)
      }
      frame "Stop Instrument" {
        # "Pass message to Instrument Manager Loop."
        n189 = call "Enqueue Message (Single).vi"("error in (no error)"=w513, "Message Data"=w511, "Message"=w510, "Message Queue"=w509) -> ("error out"=w512:errorcluster)  [unwired: 6 in, 1 out]
        n190 = Merge Errors(w512) -> (w514:errorcluster)
      }
      frame "Instrument Started" {
        # "Build an array of all processes that will receive this message"
        # "Notify processes of update"
        # "Notify processes that the instrument is running."
        n191 = Build Array(w522, w517, w516) -> (w523:refnum<queue>[])
        n192 = for {
          tunnel: w523 -> [w527] mode=indexing
          tunnel: w520 -> [w529]
          tunnel: w521 -> [w528]
          shift-right: [w526] -> w519
          shift-left: _ -> [w524]
          n193 = call "Enqueue Message (Single).vi"("Message Data"=w528, "Message"=w529, "Message Queue"=w527) -> ("error out"=w525:errorcluster)  [unwired: 7 in, 1 out]
          n194 = Merge Errors(w525, w524) -> (w526:errorcluster)
        }
      }
      frame "Instrument Stopped" {
        # "Build an array of all processes that will receive this message"
        # "Notify processes of update"
        # "Notify processes that the instrument stopped running."
        n195 = Build Array(w530, w532) -> (w533:refnum<queue>[])
        n196 = for {
          tunnel: w533 -> [w540] mode=indexing
          tunnel: w535 -> [w542]
          tunnel: w536 -> [w541]
          shift-right: [w539] -> w534
          shift-left: _ -> [w537]
          n197 = call "Enqueue Message (Single).vi"("Message Data"=w541, "Message"=w542, "Message Queue"=w540) -> ("error out"=w538:errorcluster)  [unwired: 7 in, 1 out]
          n198 = Merge Errors(w538, w537) -> (w539:errorcluster)
        }
      }
      frame "Report" {
        # "Send instrument state notification"
        # "Notify processes that the instrument stopped running."
        n199 = Variant To Data(type=T2 {"VISA Resource"="", "Setpoint"=0.0, "Running"=FALSE, "Running Since"=timestamp(0 s since 1904-01-01), "Data Point"={"Time Stamp"=timestamp(0 s since 1904-01-01), "Value"=0.0}, "Current Temperature"=0.0, "Sampling Rate (sec/sample)"=0.0} ("Instrument State"), Variant=w552) -> (data=w548:T2)  [unwired: 1 in, 1 out]
        n200 = local read "Sampling rate\n(sec/sample)"() -> (w544:dbl)
        n201 = Bundle By Name(cluster=w548, "Sampling Rate (sec/sample)"=w544) -> (w543:T2)
        n202 = Enqueue Element(queue=w549, element=w543) -> (error out=w546:errorcluster)  [unwired: 2 in, 2 out]
        n203 = Send Notification(notification=w543, notifier=w553) -> (error out=w550:errorcluster)  [unwired: 1 in, 1 out]
        n204 = Merge Errors(w546, w550) -> (w547:errorcluster)
        n205 = call "Enqueue Message (Single).vi"("Message Data"=w543, "Message"=w557, "Message Queue"=w555) -> ("error out"=w545:errorcluster)  [unwired: 7 in, 1 out]
        n206 = Merge Errors(w545, w547) -> (w556:errorcluster)
      }
    }
    n207 = call "Error Handler - System Control Loop.vi"("error in (no error)"=w250, "Message Queue"=w252) -> ("dup error in"=w251:errorcluster)  [unwired: 8 in, 1 out]
  }
  n208 = call "Instrument Manager Loop.vi"("System Control"=w4, "Instrument Manager"=w32) -> ("error out"=w17:errorcluster)  [unwired: 9 in]
  n209 = call "Logging Message Loop.vi"("System Control"=w4, "Data Queue"=w6, "Logging"=w31) -> ("error out"=w16:errorcluster)  [unwired: 8 in]
  n210 = Unregister For Events(event registration refnum=w23) -> (error out=w18:errorcluster)  [unwired: 1 in]
  n211 = Merge Errors(w27, w19, w18, w17, w16, w15, w14) -> (w12:errorcluster)
  n212 = call <vilib>:"Simple Error Handler.vi"("error in (no error)"=w12) -> ()  [unwired: 4 in, 5 out]
  n213 = Cluster To Array(cluster=w11) -> (array=w10:refnum<queue>[])
  n214 = for {
    shift-right: [w559] -> w9
    shift-left: w12 -> [w560]
    tunnel: w10 -> [w561] mode=indexing
    n215 = Release Queue(queue=w561, force destroy? (F)=TRUE, error in (no error)=w560) -> (error out=w559:errorcluster)  [unwired: 2 out]
  }
  n216 = call "Destroy User Event - Stop.vi"("error in (no error)"=w9, "User Event - Stop"=w22) -> ("error out"=w24:errorcluster)  [unwired: 9 in]
  n217 = disable-structure shown="RUN_TIME_ENGINE==True" {
    disable-tunnel: w24 -> [_ _]
    frame condition #0 (active) {
    }
    frame condition #1 {
      # "Call Quit LabVIEW if running as a built application."
      n218 = Quit LabVIEW() -> ()  [unwired: 1 in]
    }
  }
